vi "SendSinglePacket.vi"(8 "error in (no error)":errorcluster, 10 "Transmit":T1, 11 "VISA resource name":refnum<visa-resource-name>) -> (0 "error out":errorcluster, 2 "element":T1, 3 "VISA resource name out":refnum<visa-resource-name>)   [LabVIEW 2009]
uses:
  Packet.ctl
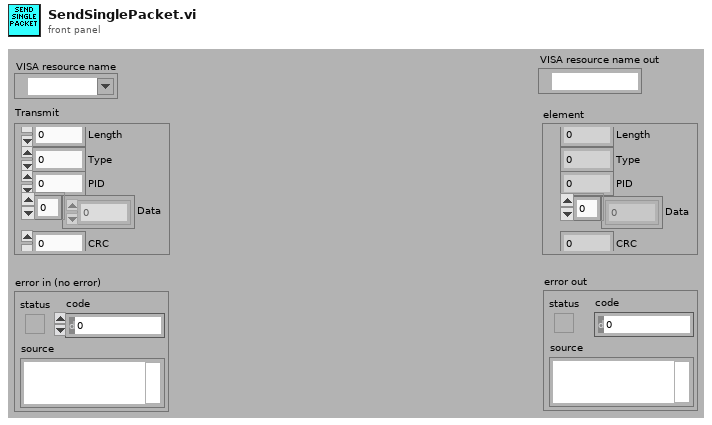
[diagram p1: front panel]
types:
  T1 = typedef "Packet.ctl" = cluster{"Length":u8, "Type":u8, "PID":u8, "Data":u8[], "CRC":u8}
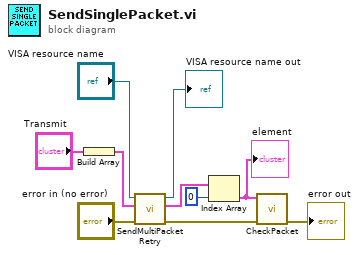
[diagram p0: block diagram]
diagram:
  n1 = Build Array("Transmit") -> (w8:T1[])
  n2 = call "SendMultiPacketRetry.vi"("error in (no error)"="error in (no error)", "Packets In"=w8, "VISA resource name"="VISA resource name") -> ("error out"=w2:errorcluster, "Packets Out"=w5:T1[], "VISA resource name 2"=→"VISA resource name out":refnum<visa-resource-name>)  [unwired: 5 in, 1 out]
  n3 = Index Array(array=w5, index=0) -> (element=w3:T1)
  "element" <- w3
  n4 = call "CheckPacket.vi"("error in"=w2, "Received"=w3) -> ("error out"=→"error out":errorcluster)  [unwired: 9 in]
